vi "Configure Waveform (Pulse).vi"(0 "VISA resource name":refnum<visa-resource-name>, 1 "Configure By (Duty Cycle)":enum16{"Duty Cycle", "Pulse Width"}(ring), 2 "Duty Cycle (10 %)":i32=10 min=0 max=100, 3 "Pulse Width (100e-6 s)":dbl=0.0001 min=2e-08 max=1999.99, 5 "Amplitude (1.0 Vpp)":dbl=1.0, 7 "Frequency (1000 Hz)":dbl=1000.0, 9 "DC Offset (0.00 V)":dbl, 11 "error in (no error)":errorcluster, 12 "Pulse Transition (5e-9 s)":dbl=5e-09 min=5e-09 max=1e-07) -> (4 "VISA resource name out":refnum<visa-resource-name>, 15 "error out":errorcluster)   [LabVIEW 2017, in "Keithley 3390.lvlib"]
doc: "Sets the waveform parameters for a pulse waveform and makes it the active waveform function."
uses:
  Keithley 3390.lvlib
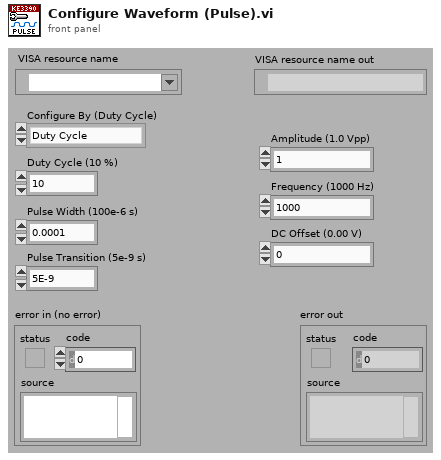
[diagram p1: front panel]
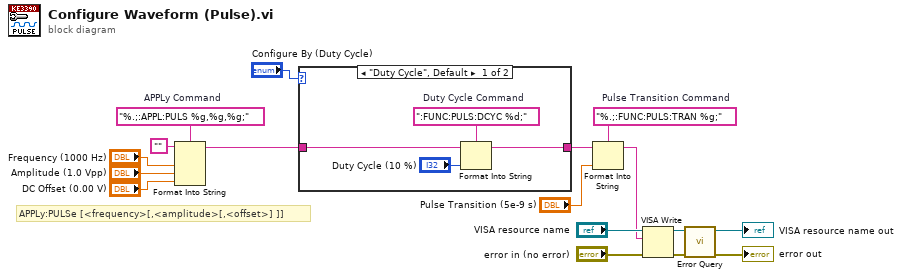
[diagram p0: block diagram]
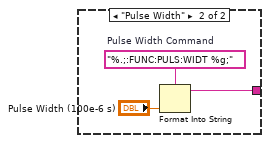
[diagram p2: hidden frame]
diagram:
  w9 = "%.;:APPL:PULS %g,%g,%g;"  # APPLy Command
  w11 = "%.;:FUNC:PULS:TRAN %g;"  # Pulse Transition Command
  # "APPLy:PULSe [<frequency>[,<amplitude>[,<offset>] ]]"
  n1 = Format Into String(format string=w9, initial string="", "Frequency (1000 Hz)", "Amplitude (1.0 Vpp)", "DC Offset (0.00 V)") -> (resulting string=w1:string)  [unwired: 1 in, 1 out]
  n2 = case shown="\"Duty Cycle\", Default" "Configure By (Duty Cycle)" {
    tunnel: [w19 w22] -> w2
    tunnel: w1 -> [w18 _]
    frame "Duty Cycle", Default {
      w20 = ":FUNC:PULS:DCYC %d;"  # Duty Cycle Command
      n3 = Format Into String(format string=w20, initial string=w18, "Duty Cycle (10 %)") -> (resulting string=w19:string)  [unwired: 1 in, 1 out]
    }
    frame "Pulse Width" {
      w23 = "%.;:FUNC:PULS:WIDT %g;"  # Pulse Width Command
      n4 = Format Into String(format string=w23, "Pulse Width (100e-6 s)") -> (resulting string=w22:string)  [unwired: 2 in, 1 out]
    }
  }
  n5 = Format Into String(format string=w11, initial string=w2, "Pulse Transition (5e-9 s)") -> (resulting string=w5:string)  [unwired: 1 in, 1 out]
  n6 = VISA Write(VISA resource name="VISA resource name", write buffer=w5, error in (no error)="error in (no error)") -> (VISA resource name out=w13:refnum<visa-resource-name>, error out=w12:errorcluster)  [unwired: 1 out]
  n7 = call "Error Query.vi"("error in (no error)"=w12, "VISA resource name"=w13) -> ("error out"=→"error out":errorcluster, "VISA resource name out"=→"VISA resource name out":refnum<visa-resource-name>)  [unwired: 6 in, 2 out]
